vi "Arduino_Close.vi"(8 "error in (no error)":errorcluster, 11 "Arduino In":T1={"Java"=path "/Applications/Arduino.app/Contents/Java", "Packages"=path "/Users/crogers/Library/Arduino15/packages", "folder"=path "/Users/crogers/Documents/LabVIEW Data", "serial"="/dev/cu.usbmodem14301", "Console"=""}) -> (0 "error out":errorcluster, 2 "Console":string)   [LabVIEW 2024]
uses:
  Arduino.ctl
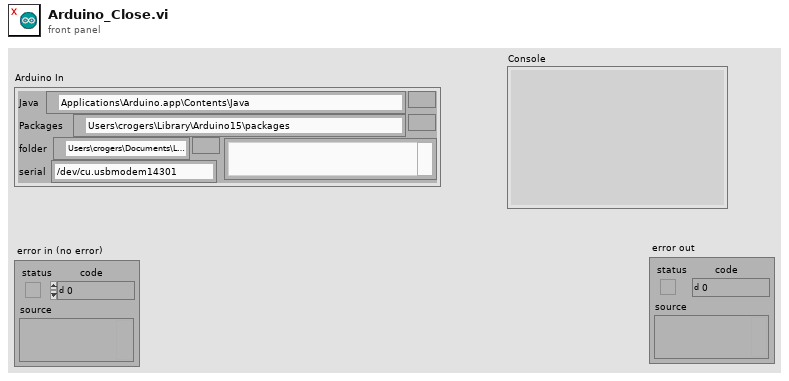
[diagram p1: front panel]
types:
  T1 = typedef "Arduino.ctl" = cluster{"Java":path, "Packages":path, "folder":path, "serial":string, "Console":string}
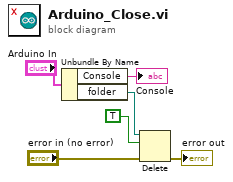
[diagram p0: block diagram]
diagram:
  n1 = Unbundle By Name("Arduino In") -> ("Console"=→"Console":string, "folder"=w6:path)
  n2 = Delete(path (use dialog)=w6, entire hierarchy (F)=TRUE, error in="error in (no error)") -> (error out=→"error out":errorcluster)  [unwired: 2 in, 2 out]
